vi "Set Result Collector.vi"(8 "error in (no error)":errorcluster, 10 "Result Collector In":refnum<class "Result Collector.lvclass">, 11 "Coverage Analyzer Process in":refnum<class "Coverage Analyzer Process.lvclass">) -> (0 "error out":errorcluster, 3 "Coverage Analyzer Process out":refnum<class "Coverage Analyzer Process.lvclass">)   [LabVIEW 2020, in "Coverage Analyzer Process.lvclass"]
uses:
  Coverage Analyzer Process.lvclass
  Coverage Analyzer Process.lvclass/Coverage Analyzer Process.ctl
  Application Framework/Process Classes/Process/Process.lvclass
  Result Collector/Result Collector.lvclass
  Result Classes/Method Result/Method Result.lvclass
  Result Classes/Test Case Result/Test Case Result.lvclass
  Result Classes/Test Suite Result/Test Suite Result.lvclass
  C:/Git/astemes-lunit/source/Application Framework/Process Classes/Process/Process.lvclass
  C:/Git/astemes-lunit/source/Framework/Coverage Analyzer Process/Coverage Analyzer Process.lvclass
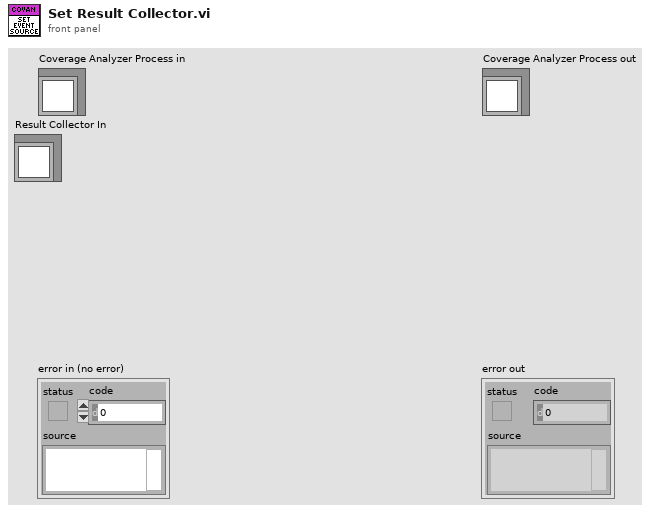
[diagram p1: front panel]
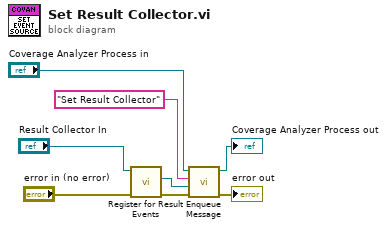
[diagram p0: block diagram]
diagram:
  n1 = call "Register for Result Events.vi"("error in (no error)"="error in (no error)", "Result Collector In"="Result Collector In") -> ("error out"=w2:errorcluster, "Event Registration Refnum"=w1:refnum<event-registration>)  [unwired: 7 in, 1 out]
  n2 = call "Enqueue Message.vi"("error in (no error)"=w2, "Message Data"=w1, "Message"="Set Result Collector", "Process In"="Coverage Analyzer Process in") -> ("error out"=→"error out":errorcluster, "Process Out"=→"Coverage Analyzer Process out":refnum<class "Coverage Analyzer Process.lvclass">)  [unwired: 6 in]
